vi "Write Word Over 2 Addresses.vi"(7 "Address number (0)":u8, 8 "error in (no error)":errorcluster, 9 "Parameter (0)":u8, 10 "Motor ID (0)":u8, 11 "Dynamixel Motor VISA in":refnum<class "Dynamixel Motor VISA.lvclass">) -> (0 "error out":errorcluster, 3 "Dynamixel Motor VISA out":refnum<class "Dynamixel Motor VISA.lvclass">)   [LabVIEW 2016, in "Dynamixel Motor VISA.lvclass"]
doc: "Writes a U8 to one address of the register on the motor. This is a Low-Level VI that is used by other VIs."
uses:
  <instrlib>/Dynamixel Motor/HAIOL/VISA/Dynamixel Motor VISA.lvclass
  <instrlib>/Dynamixel Motor/HAIOL/VISA/Dynamixel Motor VISA.lvclass/Dynamixel Motor VISA.ctl
  <instrlib>/Dynamixel Motor/Dynamixel Motor.lvlib
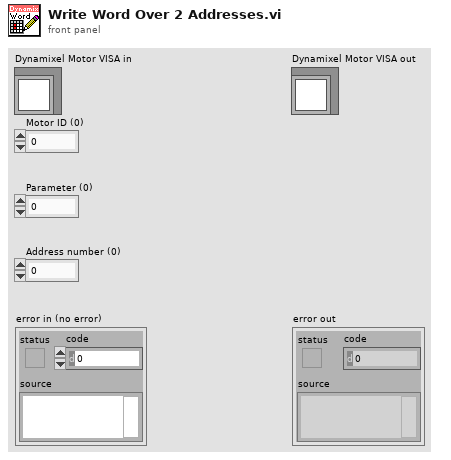
[diagram p1: front panel]
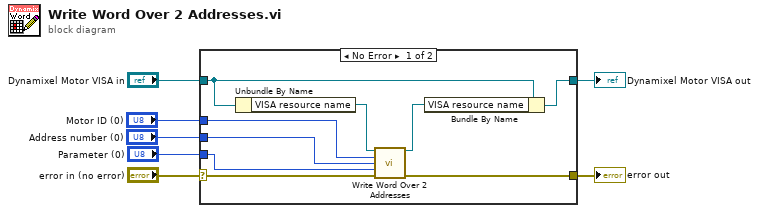
[diagram p0: block diagram]
diagram:
  n1 = case shown="No Error" "error in (no error)" {
    selector: "error in (no error)" -> [w16 w17]
    tunnel: "Dynamixel Motor VISA in" -> [w10 w18]
    tunnel: "Motor ID (0)" -> [w15 _]
    tunnel: "Parameter (0)" -> [w13 _]
    tunnel: "Address number (0)" -> [w12 _]
    tunnel: [w9 w18] -> w2
    tunnel: [w8 w17] -> w1
    frame No Error {
      n2 = Unbundle By Name(w10) -> ("VISA resource name"=w14:refnum<visa-resource-name>)
      n3 = call <instrlib>:"Write Word Over 2 Addresses.vi"("VISA resource name"=w14, "Motor ID (0)"=w15, "Address number (0)"=w12, "Parameter (0)"=w13, "error in (no error)"=w16) -> ("VISA resource name out"=w11:refnum<visa-resource-name>, "error out"=w8:errorcluster)  [unwired: 9 in]
      n4 = Bundle By Name(cluster=w10, "VISA resource name"=w11) -> (w9:refnum<class "Dynamixel Motor VISA.lvclass">)
    }
    frame Error {
    }
  }
  "error out" <- w1
  "Dynamixel Motor VISA out" <- w2
